vi "SendConfigurationToAvs47b.vi"(6 "STABILISATION DELAY (ms)":i32, 7 "WRITE ALSO TO TS-530A":bool, 8 "LV ERROR IN":errorcluster, 11 "CONFIGURATION CLUSTER":T1) -> (0 "LV ERROR OUT":errorcluster, 1 "AVS47B RXSTR":string="000000000000000000000000000000000000000000000000", 2 "AVS47B TXSTR":string="000000000000000000000011000000000000000000000000", 3 "UNMODIFIED CONFIGURATION CLUSTER":T1)   [LabVIEW 2021]
doc: "Programs the AVS-47B and optionally also\nthe TS-530A hardware."
panel:
  out "530STR":string
  # "SendConfigurationToAvs47b.vi"
  # "This VI assembles the 48-bit long binary string TXSTR, which is then sent to the AVS-47B\n(and optionally also to the TS-530A) via Picobus.  A stabilisation delay can be used for giving\nthe bridge time to find balance after a change. On the highest 3mV excitation,\n5-7 seconds would perhaps be sufficient. On the lowest 3uV excitation the bridge\nmay need over 15 seconds to find balance which is surely between the peak-to-peak\nnoise limits.  Use this VI for configuring the AVS-47B (and possibly TS-530A) before \nor if you do not need reading from the instruments. \n\nThe  ReadAvs47B.vi includes this SendConfigurationToAvs47b.vi together with\nthe stabilisation delay input. So, whenever you want also to read, use the reading VI. In cases\nwhere reading is not needed, SendConfigurationToAvs47b.vi is faster. Writing to the TS-530A\nis a very slow process, so writing should be disabled if a TS-530A is not included in the system.  \n\nDO NOT MODIFY THIS VI! It addresses the internal registers of the AVS-47B and TS-530A."
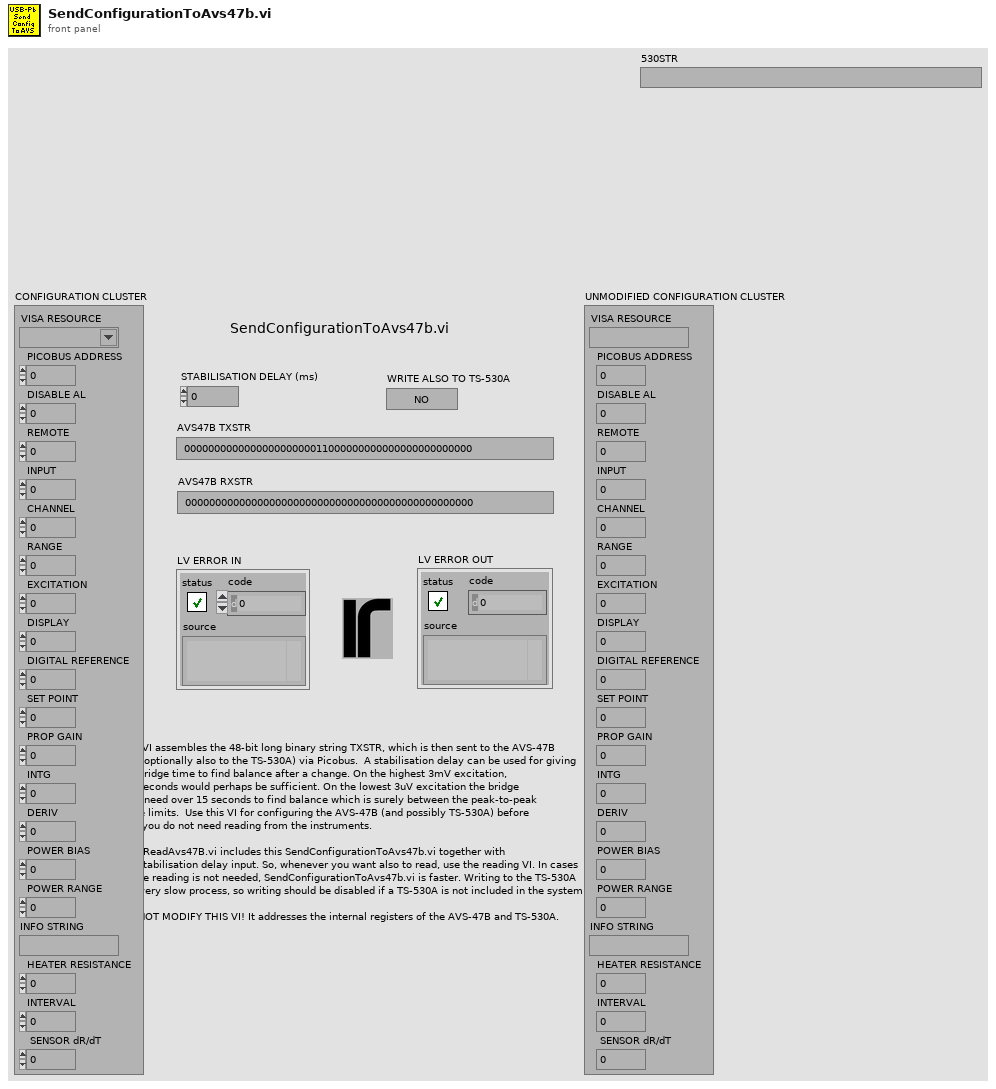
[diagram p1: front panel]
types:
  T1 = cluster{"VISA RESOURCE":refnum<visa-resource-name>, "PICOBUS ADDRESS":u8, "DISABLE AL":u8, "REMOTE":u8, "INPUT":u8, "CHANNEL":u8, "RANGE":u8, "EXCITATION":u8, "DISPLAY":u8, "DIGITAL REFERENCE":u16, "SET POINT":dbl, "PROP GAIN":u8, "INTG":u8, "DERIV":u8, "POWER BIAS":u8, "POWER RANGE":u8, "INFO STRING":string, "HEATER RESISTANCE":dbl, "INTERVAL":u8, " SENSOR dR/dT":u8}
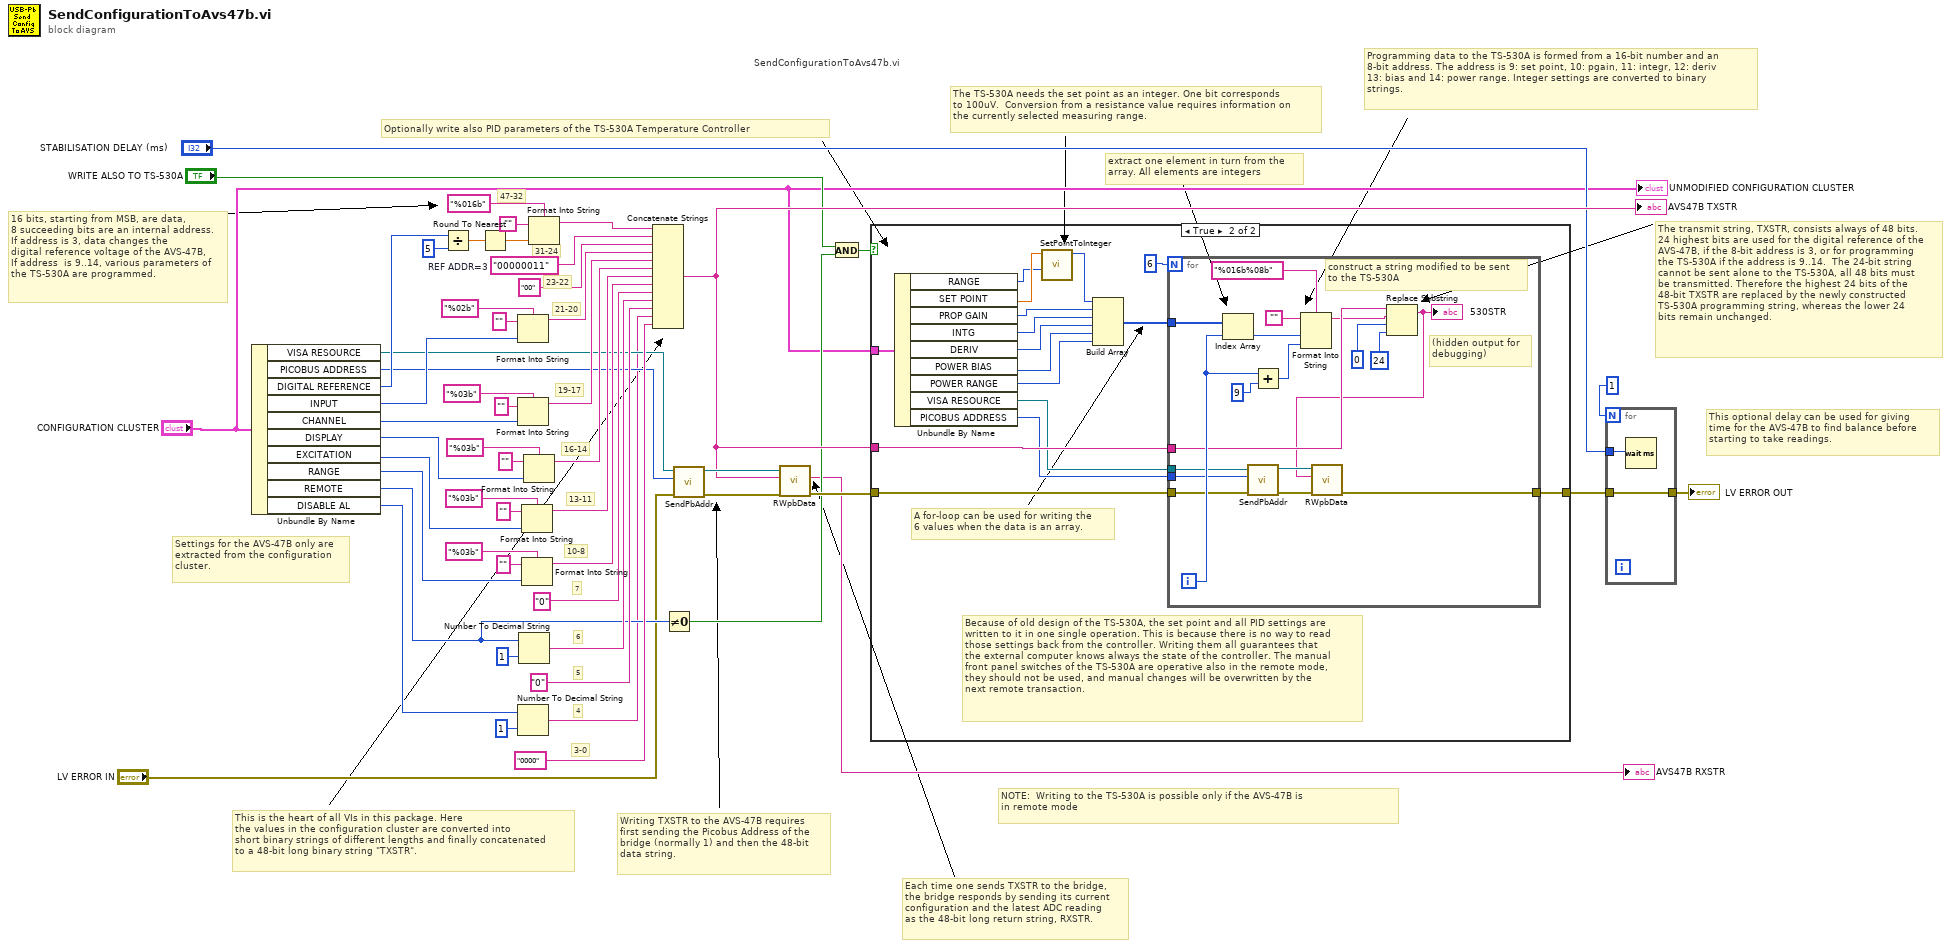
[diagram p0: block diagram]
diagram:
  w37 = "00000011"  # REF ADDR=3
  # "3-0"
  # "4"
  # "5"
  # "6"
  # "7"
  # "10-8"
  # "13-11"
  # "16-14"
  # "19-17"
  # "21-20"
  # "23-22"
  # "31-24"
  # "47-32"
  # "16 bits, starting from MSB, are data,\n8 succeeding bits are an internal address.\nIf address is 3, data changes the\ndigital reference voltage of the AVS-47B,\nIf address  is 9..14, various parameters of\nthe TS-530A are programmed."
  # "This optional delay can be used for giving\ntime for the AVS-47B to find balance before\nstarting to take readings."
  # "The transmit string, TXSTR, consists always of 48 bits.\n24 highest bits are used for the digital reference of the\nAVS-47B, if the 8-bit address is 3, or for programming\nthe TS-530A if the address is 9..14.  The 24-bit string\ncannot be sent alone to the TS-530A, all 48 bits must\nbe transmitted. Therefore the highest 24 bits of the \n48-bit TXSTR are replaced by the newly constructed\nTS-530A programming string, whereas the lower 24\nbits remain unchanged."
  # "Programming data to the TS-530A is formed from a 16-bit number and an\n8-bit address. The address is 9: set point, 10: pgain, 11: integr, 12: deriv\n13: bias and 14: power range. Integer settings are converted to binary\nstrings."
  # "extract one element in turn from the array. All elements are integers"
  # "The TS-530A needs the set point as an integer. One bit corresponds\nto 100uV.  Conversion from a resistance value requires information on\nthe currently selected measuring range."
  # "Each time one sends TXSTR to the bridge,\nthe bridge responds by sending its current\nconfiguration and the latest ADC reading\nas the 48-bit long return string, RXSTR."
  # "Writing TXSTR to the AVS-47B requires\nfirst sending the Picobus Address of the\nbridge (normally 1) and then the 48-bit\ndata string."
  # "This is the heart of all VIs in this package. Here\nthe values in the configuration cluster are converted into\nshort binary strings of different lengths and finally concatenated\nto a 48-bit long binary string \"TXSTR\"."
  # "Settings for the AVS-47B only are\nextracted from the configuration\ncluster."
  # "NOTE:  Writing to the TS-530A is possible only if the AVS-47B is\nin remote mode"
  # "SendConfigurationToAvs47b.vi"
  # "Optionally write also PID parameters of the TS-530A Temperature Controller"
  n1 = Unbundle By Name("CONFIGURATION CLUSTER") -> ("VISA RESOURCE"=w18:refnum<visa-resource-name>, "PICOBUS ADDRESS"=w19:u8, "DIGITAL REFERENCE"=w38:u16, "INPUT"=w35:u8, "CHANNEL"=w34:u8, "DISPLAY"=w33:u8, "EXCITATION"=w32:u8, "RANGE"=w31:u8, "REMOTE"=w15:u8, "DISABLE AL"=w4:u8)
  n2 = Divide(x=w38, y=5) -> (x/y=w43:dbl)
  n3 = Round To Nearest(number=w43) -> (nearest integer value=w39:dbl)
  n4 = Format Into String(format string="%02b", initial string="", w35) -> (resulting string=w30:string)  [unwired: 1 in, 1 out]
  n5 = Format Into String(format string="%03b", initial string="", w34) -> (resulting string=w29:string)  [unwired: 1 in, 1 out]
  n6 = Number To Decimal String(number=w4, width (-)=i16 1) -> (decimal integer string=w5:string)
  n7 = Number To Decimal String(number=w15, width (-)=i16 1) -> (decimal integer string=w24:string)
  n8 = Format Into String(format string="%03b", initial string="", w32) -> (resulting string=w27:string)  [unwired: 1 in, 1 out]
  n9 = Format Into String(format string="%03b", initial string="", w31) -> (resulting string=w26:string)  [unwired: 1 in, 1 out]
  n10 = Format Into String(format string="%03b", initial string="", w33) -> (resulting string=w28:string)  [unwired: 1 in, 1 out]
  n11 = Format Into String(format string="%016b", initial string="", w39) -> (resulting string=w2:string)  [unwired: 1 in, 1 out]
  n12 = Concatenate Strings(w2, w37, "00", w30, w29, w28, w27, w26, "0", w24, "0", w5, "0000") -> (w16:string)
  "AVS47B TXSTR" <- w16
  n13 = Not Equal To 0?(x=w15) -> (x != 0?=w12:bool)
  n14 = call "SendPbAddr.vi"("error in (no error)"="LV ERROR IN", "PICOBUS ADDRESS"=w19, "VISA resource"=w18) -> ("error out"=w20:errorcluster, "dup VISA resource"=w21:refnum<visa-resource-name>)  [unwired: 6 in]
  n15 = call "RWpbData.vi"("error in (no error)"=w20, "TXSTR"=w16, "VISA resource"=w21) -> ("error out"=w17:errorcluster, "RXSTR"=→"AVS47B RXSTR":string)  [unwired: 2 in, 1 out]
  n16 = And(x="WRITE ALSO TO TS-530A", y=w12) -> (x .and. y?=w14:bool)
  n17 = case shown="True" w14 {
    tunnel: w17 -> [w55 w62]
    tunnel: [w55 w70] -> w9
    tunnel: "CONFIGURATION CLUSTER" -> [_ w69]
    tunnel: w16 -> [_ w61]
    frame False {
      # "If there is no TS-530A Temperature Controller connected to \nthe resistance bridge, this case is run. Writing to the \ntemperature controller is a very slow process, therefore it \nshould be disabled if there is no controller in the system."
    }
    frame True {
      # "A for-loop can be used for writing the\n6 values when the data is an array."
      # "Because of old design of the TS-530A, the set point and all PID settings are\nwritten to it in one single operation. This is because there is no way to read\nthose settings back from the controller. Writing them all guarantees that\nthe external computer knows always the state of the controller. The manual\nfront panel switches of the TS-530A are operative also in the remote mode,\nthey should not be used, and manual changes will be overwritten by the \nnext remote transaction."
      n18 = Unbundle By Name(w69) -> ("RANGE"=w57:u8, "SET POINT"=w58:dbl, "PROP GAIN"=w68:u8, "INTG"=w67:u8, "DERIV"=w66:u8, "POWER BIAS"=w65:u8, "POWER RANGE"=w64:u8, "VISA RESOURCE"=w60:refnum<visa-resource-name>, "PICOBUS ADDRESS"=w59:u8)
      n19 = call "SetPointToInteger.vi"("RANGE"=w57, "SP OHMS"=w58) -> ("SP INTEGER"=w56:u16)  [unwired: 9 in]
      n20 = Build Array(w56, w68, w67, w66, w65, w64) -> (w63:u16[])
      n21 = for {
        N: 6 -> [_]
        tunnel: w63 -> [w89]
        tunnel: w61 -> [w84]
        tunnel: [w75] -> w70
        tunnel: w62 -> [w74]
        tunnel: w60 -> [w73]
        tunnel: w59 -> [w72]
        i -> [w87]
        # "construct a string modified to be sent\nto the TS-530A"
        # "(hidden output for\ndebugging)"
        n22 = Index Array(array=w89, index=w87) -> (element=w82:u16)
        n23 = call "SendPbAddr.vi"("error in (no error)"=w74, "PICOBUS ADDRESS"=w72, "VISA resource"=w73) -> ("error out"=w77:errorcluster, "dup VISA resource"=w78:refnum<visa-resource-name>)  [unwired: 6 in]
        n24 = Add(x=w87, y=9) -> (x+y=w81:i32)
        n25 = Format Into String(format string="%016b%08b", initial string="", w82, w81) -> (resulting string=w80:string)  [unwired: 1 in, 1 out]
        n26 = Replace Substring(2:24, 3:0, 4:w80, 5:w84) -> (1:w76:string)  [unwired: 1 out]
        "530STR" <- w76
        n27 = call "RWpbData.vi"("error in (no error)"=w77, "TXSTR"=w76, "VISA resource"=w78) -> ("error out"=w75:errorcluster)  [unwired: 2 in, 2 out]
      }
    }
  }
  n28 = for {
    N: 1 -> [_]
    tunnel: "STABILISATION DELAY (ms)" -> [w90]
    tunnel: w9 -> [w91]
    tunnel: [w91] -> w8
    n29 = Wait (ms)(milliseconds to wait=w90) -> ()  [unwired: 1 out]
  }
  "LV ERROR OUT" <- w8
  "UNMODIFIED CONFIGURATION CLUSTER" <- "CONFIGURATION CLUSTER"
